vi "Page_Version_Initialize.vi"(6 "output cluster":T1, 8 "error in (no error)":errorcluster, 11 "AB_SourceDist in":refnum<class "AB_SourceDistribution.lvclass">) -> (0 "error out":errorcluster, 3 "AB_SourceDist out":refnum<class "AB_SourceDistribution.lvclass">)   [LabVIEW 2020, in "AB_SourceDistribution.lvclass"]
uses:
  <vilib>/AppBuilder/AB_Classes/SourceDistribution/AB_SourceDistribution.lvclass
  <resource>/Framework/Providers/Builds/AppBuilder/AB_UI_Page_Version_References.ctl
  <vilib>/AppBuilder/AB_Classes/Build/AB_Build.lvclass
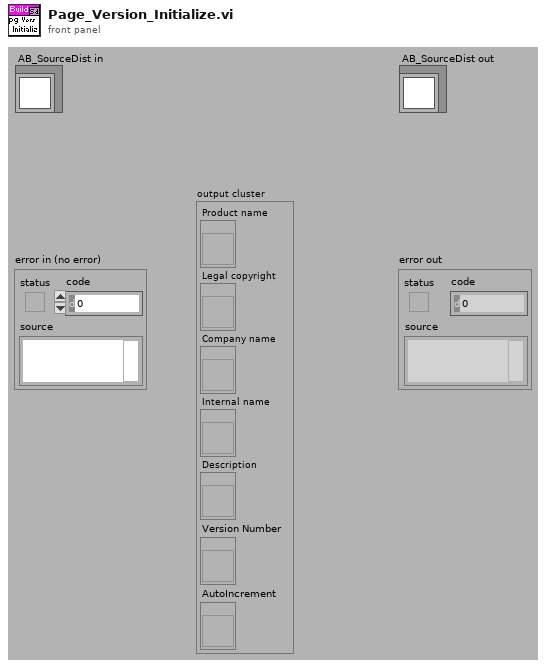
[diagram p1: front panel]
types:
  T1 = typedef "AB_UI_Page_Version_References.ctl" = cluster{"Product name":refnum<vi>, "Legal copyright":refnum<vi>, "Company name":refnum<vi>, "Internal name":refnum<vi>, "Description":refnum<vi>, "Version Number":refnum<vi>, "AutoIncrement":refnum<vi>}
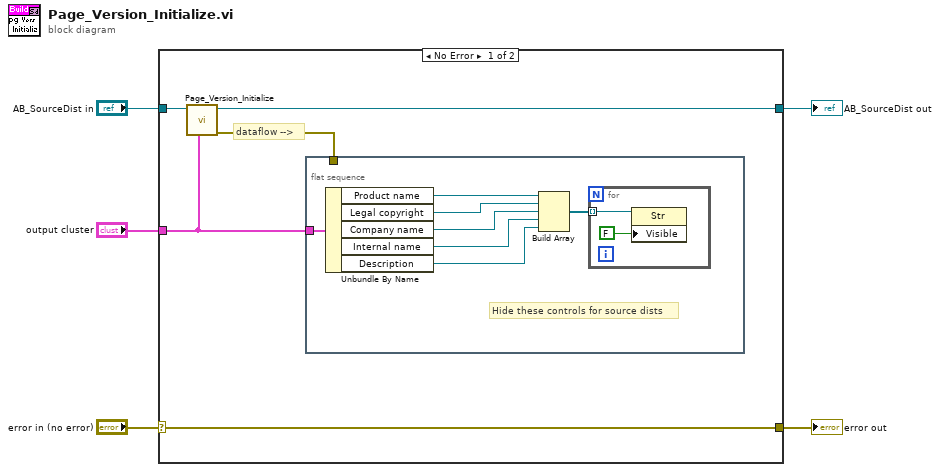
[diagram p0: block diagram]
diagram:
  n1 = case shown="No Error" "error in (no error)" {
    selector: "error in (no error)" -> [w10 w21]
    tunnel: [w10 w21] -> w2
    tunnel: [w8 w20] -> w4
    tunnel: "AB_SourceDist in" -> [w9 w20]
    tunnel: "output cluster" -> [w7 _]
    frame No Error {
      # "dataflow -->"
      n2 = call-parent "Page_Version_Initialize.vi"("output cluster"=w7, "AB_Build in"=w9) -> ("error out"=w6:errorcluster, "AB_Build out"=w8:refnum<class "AB_SourceDistribution.lvclass">)  [unwired: 8 in]
      n3 = flat-sequence {
        tunnel: w7 -> [w11]
        tunnel: w6 -> [_]
        frame #0 {
          # "Hide these controls for source dists"
          n4 = Unbundle By Name(w11) -> ("Product name"=w17:refnum<vi>, "Legal copyright"=w15:refnum<vi>, "Company name"=w14:refnum<vi>, "Internal name"=w13:refnum<vi>, "Description"=w16:refnum<vi>)
          n5 = Build Array(w17, w15, w14, w13, w16) -> (w12:refnum<vi>[])
          n6 = for {
            tunnel: w12 -> [w18] mode=indexing
            n7 = property class="Str"(reference=w18, "Visible"=FALSE) -> ()  [unwired: 1 in, 2 out]
          }
        }
      }
    }
    frame Error {
    }
  }
  "error out" <- w2
  "AB_SourceDist out" <- w4
